vi "SCLN_CheckShutdown.vi"() -> (0 "Shutdown":bool)   [LabVIEW 2015]
doc: "Check for Shutdown request.\nReturns TRUE if yes."
uses:
  SCLN_RW_Select.ctl
  SCLN_NOTIF_Select.ctl
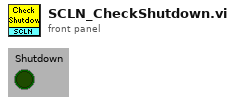
[diagram p1: front panel]
types:
  T1 = typedef "SCLN_NOTIF_Select.ctl" = enum16{"Server1", "Server2", "Server3", "Server4", "Server5", "Server6", "Server7", "Client1", "Client2", "Client3", "Client4", "Client5", "Client6", "Client7", "Client8", "Client9", "Client10", "Shutdown", "Init_Ready"}
  T2 = typedef "SCLN_RW_Select.ctl" = enum16{"Read", "Write"}
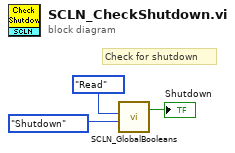
[diagram p0: block diagram]
diagram:
  # "Check for shutdown"
  n1 = call "SCLN_GlobalBooleans.vi"("Element"=SCLN_NOTIF_Select."Shutdown" ("Dome String Ctrl"), "Operation"=SCLN_RW_Select."Read" ("GBL_RW")) -> ("Read Value"=→"Shutdown":bool)  [unwired: 2 in, 1 out]
